vi "min-max-y-cursors-2D.vi"(0 "round":bool=TRUE, 1 "GRAPH EXPERIMENTAL DATA ref":refnum<vi>) -> (2 "minY":i32, 3 "maxY":i32, 4 "minX":i32, 5 "maxX":i32)   [LabVIEW 2019]
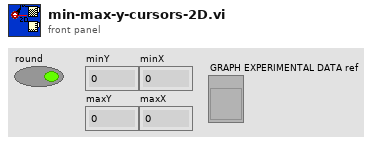
[diagram p1: front panel]
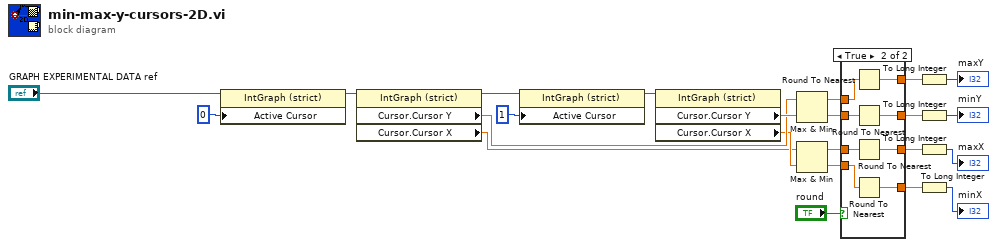
[diagram p0: block diagram]
diagram:
  n1 = property class="IntGraph (strict)"(reference="GRAPH EXPERIMENTAL DATA ref", "Active Cursor"=u32 0) -> (reference out=w17:refnum<vi>)  [unwired: 1 in, 1 out]
  n2 = property class="IntGraph (strict)"(reference=w17) -> (reference out=w18:refnum<vi>, "Cursor.Cursor Y"=w22:dbl, "Cursor.Cursor X"=w15:dbl)  [unwired: 1 in, 1 out]
  n3 = property class="IntGraph (strict)"(reference=w18, "Active Cursor"=u32 1) -> (reference out=w19:refnum<vi>)  [unwired: 1 in, 1 out]
  n4 = property class="IntGraph (strict)"(reference=w19) -> ("Cursor.Cursor Y"=w23:dbl, "Cursor.Cursor X"=w16:dbl)  [unwired: 1 in, 2 out]
  n5 = Max & Min(x=w22, y=w23) -> (max(x,y)=w11:dbl, min(x,y)=w9:dbl)
  n6 = Max & Min(x=w15, y=w16) -> (max(x,y)=w7:dbl, min(x,y)=w5:dbl)
  n7 = case shown="True" "round" {
    tunnel: [w27 w34] -> w12
    tunnel: w11 -> [w27 w35]
    tunnel: [w26 w32] -> w10
    tunnel: w9 -> [w26 w33]
    tunnel: [w25 w30] -> w8
    tunnel: w7 -> [w25 w31]
    tunnel: [w24 w28] -> w6
    tunnel: w5 -> [w24 w29]
    frame False {
    }
    frame True {
      n8 = Round To Nearest(number=w35) -> (nearest integer value=w34:dbl)
      n9 = Round To Nearest(number=w33) -> (nearest integer value=w32:dbl)
      n10 = Round To Nearest(number=w31) -> (nearest integer value=w30:dbl)
      n11 = Round To Nearest(number=w29) -> (nearest integer value=w28:dbl)
    }
  }
  n12 = To Long Integer(number=w12) -> (32bit integer=→"maxY":i32)
  n13 = To Long Integer(number=w10) -> (32bit integer=→"minY":i32)
  n14 = To Long Integer(number=w8) -> (32bit integer=→"maxX":i32)
  n15 = To Long Integer(number=w6) -> (32bit integer=→"minX":i32)
